vi "start_py.vi"(4 "error in":errorcluster) -> (0 "error out":errorcluster, 2 "Python session":refnum<k35>)   [LabVIEW 2022 SP3]
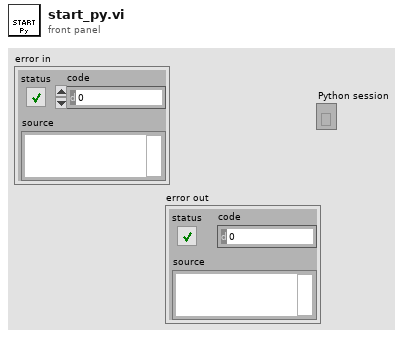
[diagram p1: front panel]
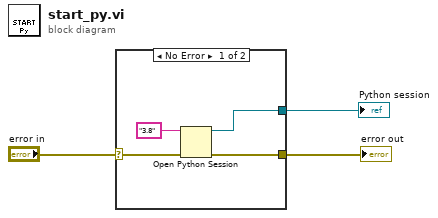
[diagram p0: block diagram]
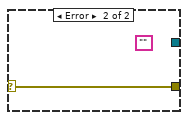
[diagram p2: hidden frame]
diagram:
  n1 = case shown="No Error" "error in" {
    selector: "error in" -> [w5 w8]
    tunnel: [w6 w8] -> w2
    tunnel: [w4 _] -> w1
    frame No Error {
      n2 = Open Python Session(python version="3.8" ("Python version"), 3:w5) -> (session out=w4:refnum<k35>, error out=w6:errorcluster)  [unwired: 1 in]
    }
    frame Error {
      (unwired) ""
    }
  }
  "error out" <- w2
  "Python session" <- w1
